vi "Velocity Drive.vi"(8 "error in (no error)":errorcluster, 9 "Right Speed":dbl, 10 "Left Speed":dbl, 11 "TalonSRX in":refnum<class "TalonSRX.lvclass">) -> (0 "error out":errorcluster, 3 "TalonSRX out":refnum<class "TalonSRX.lvclass">)   [LabVIEW 2019]
doc: "switches into velocity drive"
uses:
  TalonSRX.lvclass
  C:/Users/rishi/OneDrive/Documents/2020InfinteRecharge/src robot/Classes/Drive/Tank Drive/Tank Drive.lvclass
  <vilib>/Rock Robotics/WPI/ThirdParty/Phoenix-LabVIEW/Motor Controller/Controls/CTRE_Phoenix_MotorControl_ControlMode.ctl
  CTRE Drive.lvclass
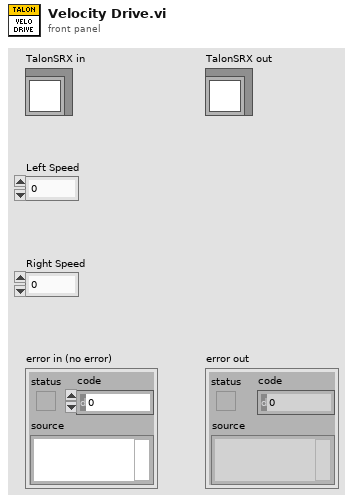
[diagram p1: front panel]
types:
  T1 = typedef "CTRE_Phoenix_MotorControl_ControlMode.ctl" = u16
  T2 = typedef "WPI_MotorControlDeviceRef.ctl" = cluster{"DeviceStatus":errorcluster, "Type":T3, "PWM":cluster{"PWM Channel":T4, "DeadBand":T5}, "CAN":cluster{"Device Number":u8, "SetOutput VI Ref":variant, "GetOutput VI Ref":variant, "Enable VI Ref":variant, "Disable VI Ref":variant, "Data":variant}, "Invert":bool, "DIO PWM":cluster{"PWM \"Enable\" Channel":T4, "DIOChannel":T6, "PWM Rate":dbl}}
  T3 = typedef "WPI_MotorControlType.ctl" = enum16{"PWM", "CAN", "DIO PWM"}
  T4 = typedef "FPGA_DIOPWMChannel.ctl" = enum8{"PWM 0", "PWM 1", "PWM 2", "PWM 3", "PWM 4", "PWM 5", "PWM 6", "PWM 7", "PWM 8", "PWM 9", "PWM MXP 0", "PWM MXP 1", "PWM MXP 2", "PWM MXP 3", "PWM MXP 4", "PWM MXP 5", "PWM MXP 6", "PWM MXP 7", "PWM MXP 8", "PWM MXP 9", "Invalid"}
  T5 = typedef "WPI_PWMDeadband.ctl" = cluster{"Name":string, "maxPositivePwm":i32, "minPositivePwm":i32, "centerPwm":i32, "maxNegativePwm":i32, "minNegativePwm":i32, "angularRange":u16}
  T6 = typedef "FPGA_DIOChannel.ctl" = enum8{"DIO 0", "DIO 1", "DIO 2", "DIO 3", "DIO 4", "DIO 5", "DIO 6", "DIO 7", "DIO 8", "DIO 9", "DIO MXP 0", "DIO MXP 1", "DIO MXP 2", "DIO MXP 3", "DIO MXP 4", "DIO MXP 5", "DIO MXP 6", "DIO MXP 7", "DIO MXP 8", "DIO MXP 9", "DIO MXP 10", "DIO MXP 11", "DIO MXP 12", "DIO MXP 13", "DIO MXP 14", "DIO MXP 15", "SPI Port CS1", "SPI Port CS2", "SPI Port CS3", "SPI Port MISO", "SPI Port MOSI", "Invalid"}
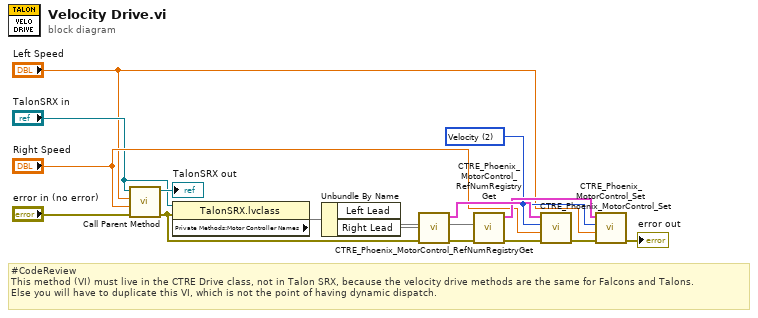
[diagram p0: block diagram]
diagram:
  w8 = T1 2 items=["PercentOutput"=0, "Position"=1, "Velocity"=2, "Current"=3, "Follower"=5, "MotionProfile"=6, "MotionMagic"=7, "MotionProfileArc"=10, "Disabled"=15] ("Control Mode")
  # "#CodeReview\nThis method (VI) must live in the CTRE Drive class, not in Talon SRX, because the velocity drive methods are the same for Falcons and Talons.\nElse you will have to duplicate this VI, which is not the point of having dynamic dispatch."
  n1 = call-parent "Call Parent Method"("error in (no error)"="error in (no error)", "Right Speed"="Right Speed", "Left Speed"="Left Speed", "CTRE Drive in"="TalonSRX in") -> ("error out"=w5:errorcluster, "CTRE Drive out"=→"TalonSRX out":refnum<class "TalonSRX.lvclass">)  [unwired: 6 in]
  n2 = property class="TalonSRX.lvclass"(reference="TalonSRX in", error in=w5) -> ("Private Methods:Motor Controller Names"=w15)  [unwired: 2 out]
  n3 = Unbundle By Name(w15) -> ("Left Lead"=w14, "Right Lead"=w13)
  n4 = call <vilib>:"CTRE_Phoenix_MotorControl_RefNumRegistryGet.vi"("error in (no error)"=w5, "refnum name"=w14) -> ("error out"=w2:errorcluster, "PhoenixMotorControlDevRef"=w11:T2)  [unwired: 8 in]
  n5 = call <vilib>:"CTRE_Phoenix_MotorControl_RefNumRegistryGet.vi"("error in (no error)"=w2, "refnum name"=w13) -> ("error out"=w9:errorcluster, "PhoenixMotorControlDevRef"=w10:T2)  [unwired: 8 in]
  n6 = call <vilib>:"CTRE_Phoenix_MotorControl_Set.vi"("error in (no error)"=w9, "Output"="Right Speed", "Control Mode"=w8, "PhoenixMotorControlDevRef"=w11) -> ("error out"=w12:errorcluster)  [unwired: 6 in, 1 out]
  n7 = call <vilib>:"CTRE_Phoenix_MotorControl_Set.vi"("error in (no error)"=w12, "Output"="Left Speed", "Control Mode"=w8, "PhoenixMotorControlDevRef"=w10) -> ("error out"=→"error out":errorcluster)  [unwired: 6 in, 1 out]
